vi "JSON Error Cluster From Error Code.vi"(6 "VI depth (1)":i32=1, 8 "error in (no error)":errorcluster, 9 "Error message":string, 10 "JSON error code":i32=8801, 11 "JSON Value in":refnum<class "JSON Value.lvclass">) -> (0 "error out":errorcluster, 3 "JSON Value out":refnum<class "JSON Value.lvclass">)   [LabVIEW 2011, in "JSON Value.lvclass"]
uses:
  JSON Value.lvclass
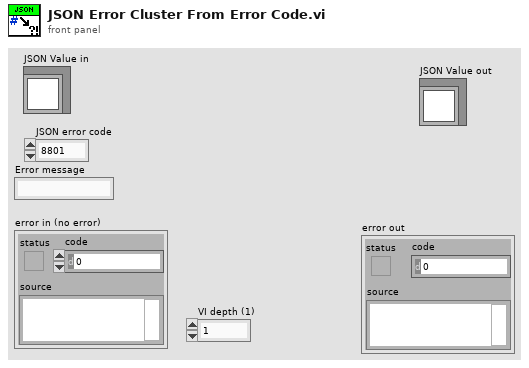
[diagram p1: front panel]
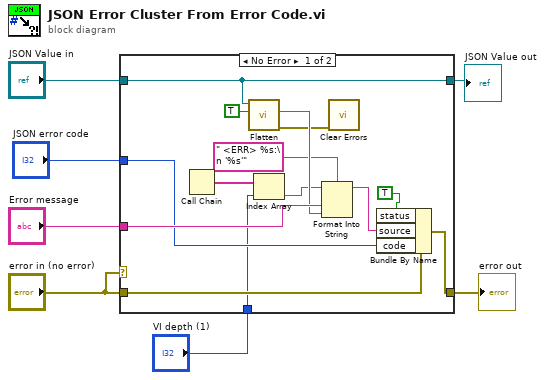
[diagram p0: block diagram]
diagram:
  n1 = case shown="No Error" "error in (no error)" {
    tunnel: "Error message" -> [w21 _]
    tunnel: "error in (no error)" -> [w19 w23]
    tunnel: "JSON error code" -> [w17 _]
    tunnel: [w10 w23] -> w5
    tunnel: "JSON Value in" -> [w9 w22]
    tunnel: [w9 w22] -> w2
    tunnel: "VI depth (1)" -> [w8 _]
    frame No Error {
      n2 = Call Chain() -> (call chain=w15:string[])
      n3 = call-dynamic "Flatten.vi"("Pretty Print?"=TRUE, "JSON Value in"=w9) -> ("error out"=w11:errorcluster, "String"=w18:string)  [unwired: 8 in]
      n4 = Index Array(array=w15, index=w8) -> (element=w14:string)
      n5 = Format Into String(format string=" <ERR> %s:\n '%s'", initial string=w14, w21, w18) -> (resulting string=w16:string)  [unwired: 1 in, 1 out]
      n6 = call <vilib>:"Clear Errors.vi"("error in (no error)"=w11) -> ()  [unwired: 6 in, 1 out]
      n7 = Bundle By Name(cluster=w19, "status"=TRUE, "source"=w16, "code"=w17) -> (w10:errorcluster)
    }
    frame Error {
    }
  }
  "error out" <- w5
  "JSON Value out" <- w2
